vi "Vibration main_solution.vi"() -> ()   [LabVIEW 2013]
uses:
  <vilib>/measure/maspectr.llb/Power Spectrum and PSD Export Mode.ctl
  <vilib>/Analysis/4window.llb/windowTd.ctl
  <vilib>/DAQmx/write.llb/DAQmx Write (Analog DBL 1Chan 1Samp).vi
  <vilib>/DAQmx/read.llb/DAQmx Read (Analog Wfm 1Chan NSamp).vi
  <vilib>/DAQmx/create/channels.llb/DAQmx Create Channel (AI-Acceleration-Accelerometer).vi
  <vilib>/DAQmx/configure/timing.llb/DAQmx Timing (Sample Clock).vi
  <vilib>/DAQmx/create/channels.llb/DAQmx Create Channel (AO-Voltage-Basic).vi
  <vilib>/measure/maspectr.llb/FFT Power Spectrum and PSD for 1 Chan.vi
  <vilib>/measure/matone.llb/Extract Single Tone Information 1 Chan.vi
  <vilib>/DAQmx/miscellaneous.llb/DAQmx Fill In Error Info.vi
  <vilib>/imath/engines/lvmath2/RunTimeEngine/ErrorHandling/NIMS_Finalize Error.vi
  <vilib>/imath/engines/lvmath2/RunTimeEngine/BuiltInFunctions/length/NIMS_length(GV).vi
  <instcachedir>/0/NIMS_length(GV)_08A3D13377FD4E4B96F5795FBF3698FA.lvgen/NIMS_length(GV)_08A3D13377FD4E4B96F5795FBF3698FA_000.vi
  <vilib>/imath/engines/lvmath2/RunTimeEngine/NodeEndStatement/NIMS_NodeEndStatement_Output.vi
  <instcachedir>/0/NIMS_NodeEndStatement_Output_53EC0D466D134D7ABD903AC30B43404B.lvgen/NIMS_NodeEndStatement_Output_53EC0D466D134D7ABD903AC30B43404B_001.vi
  <instcachedir>/0/NIMS_NodeEndStatement_Output_53EC0D466D134D7ABD903AC30B43404B.lvgen/NIMS_NodeEndStatement_Output_53EC0D466D134D7ABD903AC30B43404B_005.vi
  <vilib>/imath/engines/lvmath2/RunTimeEngine/BuiltInFunctions/fft/NIMS_fft(GV).vi
  <instcachedir>/0/NIMS_fft(GV)_4C6467FC22F84E4BA42517A07EF978B0.lvgen/NIMS_fft(GV)_4C6467FC22F84E4BA42517A07EF978B0_000.vi
  <vilib>/imath/engines/lvmath2/RunTimeEngine/ErrorHandling/NIMS_Error From Error Code.vi
  <vilib>/imath/engines/lvmath2/RunTimeEngine/BuiltInFunctions/conjugate/NIMS_conjugate(Complex).vi
  <instcachedir>/0/NIMS_conjugate(Complex)_151E186CA54B4853A0120BB0A667D86E.lvgen/NIMS_conjugate(Complex)_151E186CA54B4853A0120BB0A667D86E_001.vi
  <vilib>/imath/engines/lvmath2/RunTimeEngine/ArithmeticOperatorToken/NIMS_ArithmeticOperator_times.vi
  <instcachedir>/0/NIMS_ArithmeticOperator_times_F6527734CE75451889337B8CE94765C6.lvgen/NIMS_ArithmeticOperator_times_F6527734CE75451889337B8CE94765C6_003.vi
  <vilib>/imathl/engines/lvmath/Functions/Error Handling/Create Error.vi
  <vilib>/imath/engines/lvmath2/RunTimeEngine/RangeToken/NIMS_Range.vi
  <instcachedir>/0/NIMS_Range_7481B155BEE341ECA0F59DDB444E2C09.lvgen/NIMS_Range_7481B155BEE341ECA0F59DDB444E2C09_000.vi
  <vilib>/imath/engines/lvmath2/RunTimeSupport/NIMS_Error if Not Equal.vi
  <instcachedir>/0/NIMS_Error if Not Equal_902F5D2649E64F5087A1EF57C55C58AB.lvgen/NIMS_Error if Not Equal_902F5D2649E64F5087A1EF57C55C58AB_001.vi
  <vilib>/imath/engines/lvmath2/RunTimeEngine/IndexRead/NIMS M(S,V).vi
  <instcachedir>/0/NIMS M(S,V)_5C1965D37F59432CA0E9661793EAFE90.lvgen/NIMS M(S,V)_5C1965D37F59432CA0E9661793EAFE90_000.vi
  <vilib>/imath/engines/lvmath2/RunTimeEngine/ErrorHandling/NIMS_Create Error From Enums.vi
  <vilib>/measure/NI_MAPro.lvlib
  <vilib>/Analysis/NI_AALPro.lvlib
panel:
  out "Detected Amplitude":dbl
  out "Fan Warning":bool
  in  "Max Vib Level":dbl=0.03
  out "Detected Tone":dbl
  in  "Fan Speed Channel":tag="Voltage_out/ao1"
  in  "Tab Control":enum32{"LabVIEW PS", "MathScript PS"}(tab)
  out "PS LabVIEW":cluster{"f0":dbl, "df":dbl, "magnitude":dbl[]}(graph)={"f0"=0.0, "df"=10.240000000000004, "magnitude"=[]}
  out "PS MS":cluster{dbl, "df":dbl, "freq":dbl[]}(graph)={0.0, "df"=10.240000000000004, "freq"=[]}
  in  "Fan Speed":dbl(knob) scale=0.0..10.0
  out "Time Domain":waveform(dbl)(graph)={"t0"=timestamp(3438622544.0521445 s since 1904-01-01), "dt"=9.765624999999998e-05, "Y"=array[1000 elements], "attributes"=variant("NI_ChannelName"=variant(string "Sound_Vibration/ai0"), "NI_UnitDescription"=variant(string "g"), "NI_dBReference"=variant(dbl 1.0))}
  in  "Sample Rate":dbl=10000.0
  in  "Samples Per Channel":i32=1000
  in  "Stop Button":bool
  in  "Vibration Channel":tag="Sound_Vibration/ai0"
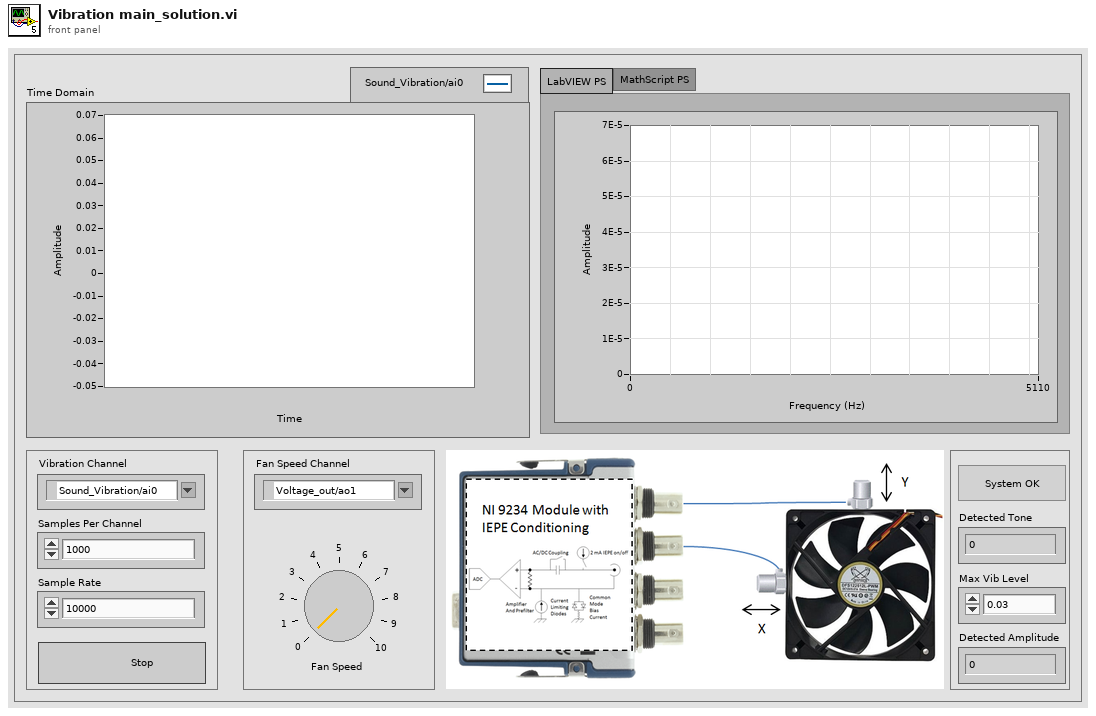
[diagram p1: front panel]
types:
  T1 = typedef "NI_AALPro.lvlib/windowTd.ctl" = u32
  T2 = typedef "NI_MAPro.lvlib/Power Spectrum and PSD Export Mode.ctl" = u16
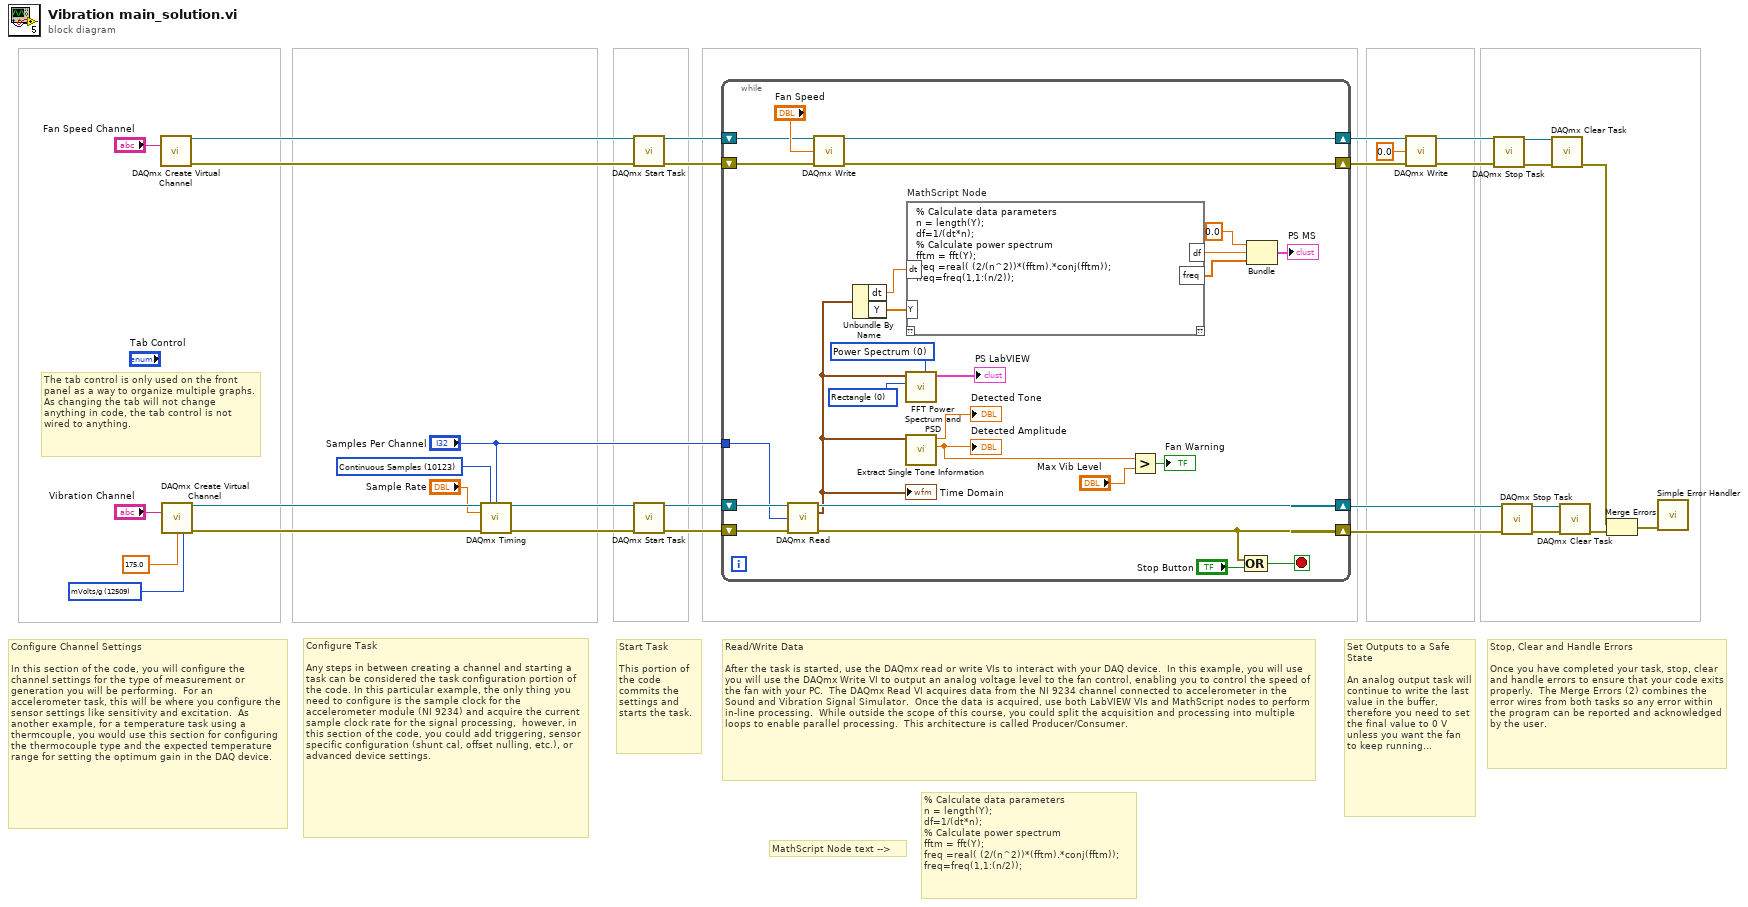
[diagram p0: block diagram]
diagram:
  w19 = 12509 items=["mVolts/g"=12509, "Volts/g"=12510] ("sensitivity units")
  w23 = 10123 items=["Finite Samples"=10178, "Continuous Samples"=10123, "Hardware Timed Single Point"=12522] ("sample mode")
  # "MathScript Node text -->"
  # "% Calculate data parameters\nn = length(Y); \ndf=1/(dt*n);\n% Calculate power spectrum\nfftm = fft(Y);\nfreq =real( (2/(n^2))*(fftm).*conj(fftm));\nfreq=freq(1,1:(n/2));"
  # "The tab control is only used on the front panel as a way to organize multiple graphs.  As changing the tab will not change anything in code, the tab control is not wired to anything."
  # "Set Outputs to a Safe State\n\nAn analog output task will continue to write the last value in the buffer, therefore you need to set the final value to 0 V unless you want the fan to keep running..."
  # "Stop, Clear and Handle Errors\n\nOnce you have completed your task, stop, clear and handle errors to ensure that your code exits properly.  The Merge Errors (2) combines the error wires from both tasks so any error within the program can be reported and acknowledged by the user."
  # "Read/Write Data\n\nAfter the task is started, use the DAQmx read or write VIs to interact with your DAQ device.  In this example, you will use you will use the DAQmx Write VI to output an analog voltage level to the fan control, enabling you to control the speed of the fan with your PC.  The DAQmx Read VI acquires data from the NI 9234 channel connected to accelerometer in the Sound and Vibration Signal Simulator.  Once the data is acquired, use both LabVIEW VIs and MathScript nodes to perform in-line processing.  While outside the scope of this course, you could split the acquisition and processing into multiple loops to enable parallel processing.  This architecture is called Producer/Consumer."
  # "Start Task\n\nThis portion of the code commits the settings and starts the task."
  # "Configure Task\n\nAny steps in between creating a channel and starting a task can be considered the task configuration portion of the code. In this particular example, the only thing you need to configure is the sample clock for the accelerometer module (NI 9234) and acquire the current sample clock rate for the signal processing,  however, in this section of the code, you could add triggering, sensor specific configuration (shunt cal, offset nulling, etc.), or advanced device settings."
  # "Configure Channel Settings\n\nIn this section of the code, you will configure the channel settings for the type of measurement or generation you will be performing.  For an accelerometer task, this will be where you configure the sensor settings like sensitivity and excitation.  As another example, for a temperature task using a thermcouple, you would use this section for configuring  the thermocouple type and the expected temperature range for setting the optimum gain in the DAQ device."
  n1 = call-poly <vilib>:"DAQmx Create Virtual Channel.vi"("physical channels"="Fan Speed Channel") -> ("task out"=w10:refnum<k21>, "error out"=w16:errorcluster)  [unwired: 13 in]
  n2 = call-poly <vilib>:"DAQmx Create Virtual Channel.vi"("physical channels"="Vibration Channel", "sensitivity"=175.0, "sensitivity units"=w19) -> ("task out"=w31:refnum<k21>, "error out"=w27:errorcluster)  [unwired: 11 in]
  n3 = call-poly <vilib>:"DAQmx Timing.vi"("task/channels in"=w31, "sample mode"=w23, "samples per channel"="Samples Per Channel", "rate"="Sample Rate", "error in"=w27) -> ("task out"=w8:refnum<k21>, "error out"=w7:errorcluster)  [unwired: 9 in]
  n4 = call <vilib>:"DAQmx Start Task.vi"("task/channels in"=w10, "error in"=w16) -> ("task out"=w9:refnum<k21>, "error out"=w17:errorcluster)  [unwired: 12 in]
  n5 = call <vilib>:"DAQmx Start Task.vi"("task/channels in"=w8, "error in"=w7) -> ("task out"=w30:refnum<k21>, "error out"=w26:errorcluster)  [unwired: 12 in]
  n6 = while {
    shift-right: [w56] -> w25
    shift-left: w26 -> [w44]
    shift-right: [w57] -> w29
    shift-left: w30 -> [w45]
    shift-right: [w51] -> w3
    shift-left: w17 -> [w52]
    shift-right: [w50] -> w6
    shift-left: w9 -> [w48]
    tunnel: "Samples Per Channel" -> [w37]
    stop <- w55 stop-if-true
    w33 = T1 0 items=["Rectangle"=0, "Hanning"=1, "Hamming"=2, "Blackman-Harris"=3, "Exact Blackman"=4, "Blackman"=5, "Flat Top"=6, "4 Term B-Harris "=7, "7 Term B-Harris"=8, "Low Sidelobe"=9, "Blackman Nuttall"=11, "Triangle"=30, "Bartlett-Hanning"=31, "Bohman"=32, "Parzen"=33, "Welch"=34, "Kaiser"=60, "Dolph-Chebyshev"=61, "Gaussian"=62] ("window")
    w43 = T2 0 items=["Power Spectrum", "Power Spectral Density"] ("export mode")
    n7 = call-poly <vilib>:"DAQmx Read.vi"("task/channels in"=w45, "number of samples per channel"=w37, "error in"=w44) -> ("task out"=w57:refnum<k21>, "data"=w42:waveform(dbl), "error out"=w56:errorcluster)  [unwired: 10 in]
    "Time Domain" <- w42
    n8 = call-poly <vilib>:"DAQmx Write.vi"("task/channels in"=w48, "data"="Fan Speed", "error in"=w52) -> ("task out"=w50:refnum<k21>, "error out"=w51:errorcluster)  [unwired: 10 in, 1 out]
    n9 = Unbundle By Name(w42) -> ("dt"=w38:dbl, "Y"=w39:dbl[])
    n10 = call-poly <vilib>:"FFT Power Spectrum and PSD.vi"("export mode"=w43, "window"=w33, "time signal"=w42) -> ("Power Spectrum / PSD"=→"PS LabVIEW":cluster{"f0":dbl, "df":dbl, "magnitude":dbl[]})  [unwired: 5 in, 3 out]
    n11 = call-poly <vilib>:"Extract Single Tone Information.vi"("time signal in"=w42) -> ("detected amplitude"=w41:dbl, "detected frequency"=→"Detected Tone":dbl)  [unwired: 5 in, 4 out]
    "Detected Amplitude" <- w41
    n12 = mathscript code="% Calculate data parameters\nn = length(Y); \ndf=1/(dt*n);\n% Calculate power spectrum\nfftm = fft(Y);\nfreq =real( (2/(n^2))*(fftm).*conj(fftm));\nfreq=freq(1,1:(n/2));"("Y"=w39, "dt"=w38) -> ("freq"=w34:dbl[], "df"=w35:dbl)  [unwired: 1 in, 1 out]
    n13 = Greater?(x=w41, y="Max Vib Level") -> (0:→"Fan Warning":bool)
    n14 = Compound Arithmetic op=OR(w56, "Stop Button") -> (w55:bool)
    n15 = Bundle(0.0, "df"=w35, "freq"=w34) -> (→"PS MS":cluster{dbl, "df":dbl, "freq":dbl[]})  [unwired: 1 in]
  }
  n16 = call-poly <vilib>:"DAQmx Write.vi"("task/channels in"=w6, "data"=0.0, "error in"=w3) -> ("task out"=w5:refnum<k21>, "error out"=w2:errorcluster)  [unwired: 10 in, 1 out]
  n17 = call <vilib>:"DAQmx Stop Task.vi"("task/channels in"=w5, "error in"=w2) -> ("task out"=w14:refnum<k21>, "error out"=w15:errorcluster)  [unwired: 12 in]
  n18 = call <vilib>:"DAQmx Stop Task.vi"("task/channels in"=w29, "error in"=w25) -> ("task out"=w28:refnum<k21>, "error out"=w24:errorcluster)  [unwired: 12 in]
  n19 = call <vilib>:"DAQmx Clear Task.vi"("task in"=w14, "error in"=w15) -> ("error out"=w13:errorcluster)  [unwired: 13 in]
  n20 = call <vilib>:"DAQmx Clear Task.vi"("task in"=w28, "error in"=w24) -> ("error out"=w12:errorcluster)  [unwired: 13 in]
  n21 = Merge Errors(w13, w12) -> (w11:errorcluster)
  n22 = call <vilib>:"Simple Error Handler.vi"("error in (no error)"=w11) -> ()  [unwired: 4 in, 5 out]
